vi "FTW-Test-SQLite-Random.vi"() -> (0 "Test Result":errorcluster)   [LabVIEW 2014]
uses:
  src/core/error/FTW-ERR-Assert-DeveloperError.vi
  src/core/error/FTW-ERR-ThrowError.vi
  src/core/error/FTW-ERR-NoErrorConstant.vi
  src/core/error/FTW-ERR-CallChain.vi
  src/core/string/FTW-STR-ReplaceWhitespace.vi
  src/core/database/FTW-SQLite-Connector.lvclass
panel:
  out "Array":string[](array[string])
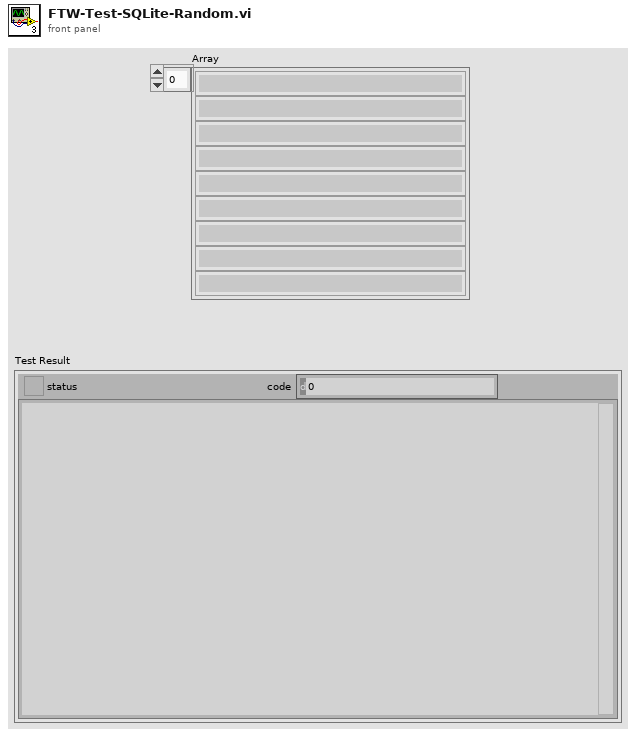
[diagram p1: front panel]
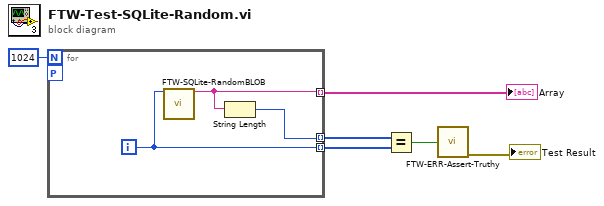
[diagram p0: block diagram]
diagram:
  n1 = for {
    N: 1024 -> [_]
    tunnel: [w7] -> w6 mode=indexing
    tunnel: [w9] -> w2 mode=indexing
    tunnel: [w8] -> w3 mode=indexing
    workers-P: _ -> [_]
    i -> [w9]
    n2 = call "FTW-SQLite-RandomBLOB.vi"("Number of Bytes"=w9) -> ("Random BLOB"=w7:string)  [unwired: 13 in, 1 out]
    n3 = String Length(string=w7) -> (length=w8:i32)
  }
  "Array" <- w6
  n4 = Equal?(x=w3, y=w2) -> (x = y?=w1:bool)
  n5 = call "FTW-ERR-Assert-Truthy.vi"("Expected Truthy"=w1) -> ("error out"=→"Test Result":errorcluster)  [unwired: 14 in]
